vi "EnableDrives.vi"(2 "error in (no error)":errorcluster, 3 "Drives to enable":string="5100,7100,7200") -> (0 "error out":errorcluster)   [LabVIEW 2009]
doc: "Closes channel for specified ID"
panel:
  out "SCPI command":string
  # "Beware: This routine resets the modules to the user default switch positions!!!"
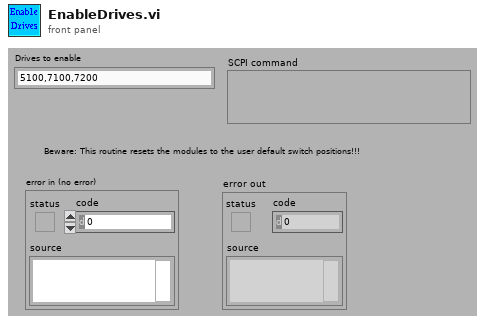
[diagram p1: front panel]
types:
  T1 = enum16{"N1911A", "Siggen", "34980a", "E4418B", "Rvp8"}
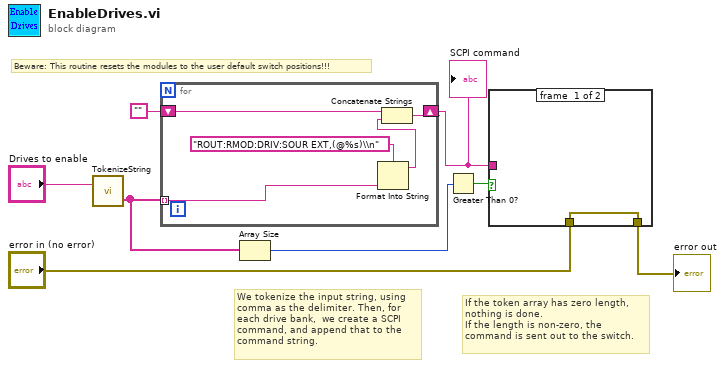
[diagram p0: block diagram]
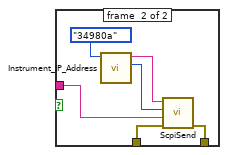
[diagram p2: hidden frame]
diagram:
  # "Beware: This routine resets the modules to the user default switch positions!!!"
  # "If the token array has zero length, nothing is done.\nIf the length is non-zero, the command is sent out to the switch."
  # "We tokenize the input string, using comma as the delimiter. Then, for each drive bank,  we create a SCPI command, and append that to the command string."
  n1 = call "TokenizeString.vi"("String to be tokenized"="Drives to enable") -> ("Output array"=w2:string[])  [unwired: 2 in]
  n2 = for {
    tunnel: w2 -> [w12] mode=indexing
    shift-right: [w11] -> w5
    shift-left: "" -> [w10]
    n3 = Format Into String(format string="ROUT:RMOD:DRIV:SOUR EXT,(@%s)\\n", w12) -> (resulting string=w9:string)  [unwired: 2 in, 1 out]
    n4 = Concatenate Strings(w10, w9) -> (w11:string)
  }
  "SCPI command" <- w5
  n5 = Array Size(array=w2) -> (size(s)=w1:i32)
  n6 = Greater Than 0?(x=w1) -> (x > 0?=w6:bool)
  n7 = case shown="True" w6 {
    tunnel: w5 -> [_ w19]
    tunnel: "error in (no error)" -> [w14 w18]
    tunnel: [w14 w17] -> w3
    frame #0 {
    }
    frame #1 {
      n8 = call "Instrument_IP_Address.vi"("Instrument"=T1."34980a") -> ("Port"=w20:u16, "IP Address"=w16:string)  [unwired: 9 in]
      n9 = call "ScpiSend.vi"("error in (no error)"=w18, "Command"=w19, "TCP port"=w20, "IP Address"=w16) -> ("error out"=w17:errorcluster)  [unwired: 7 in]
    }
  }
  "error out" <- w3
